vi "CONEX_SAG_control.vi"() -> ()   [LabVIEW 2016]
uses:
  <vilib>/Instr/_visa.llb/VISA Open Access Mode.ctl
panel:
  out "Actual Velocity [mm/s]":dbl
  out "write buffer":string
  in  "STOP":bool
  out "read buffer":string
  out "error out":errorcluster
  in  "error in (no error)":errorcluster
  in  "VISA resource name":refnum<visa-resource-name>="COM9"
  in  "Set new velocity":bool
  in  "Velocity [mm/s]":sgl=1.0
  in  "HOME":bool
  in  "Move Absolute":bool
  in  "Set Absolute Position":sgl=2.0
  in  "Move Relative":bool
  in  "Set Relative Position":sgl=1.0
  out "Current\nPosition\n[mm]":sgl=19.930592 format="%_8f"
  in  "stop code":bool
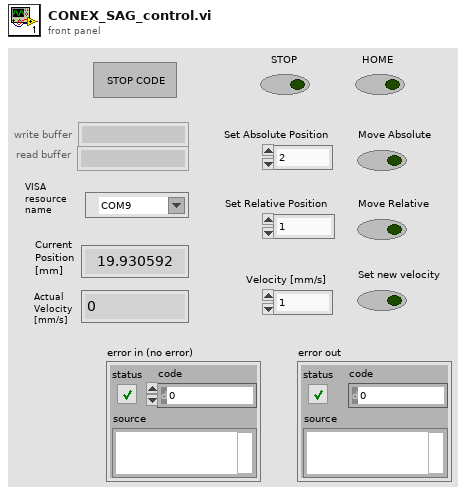
[diagram p1: front panel]
types:
  T1 = typedef "VISA Open Access Mode.ctl" = u32
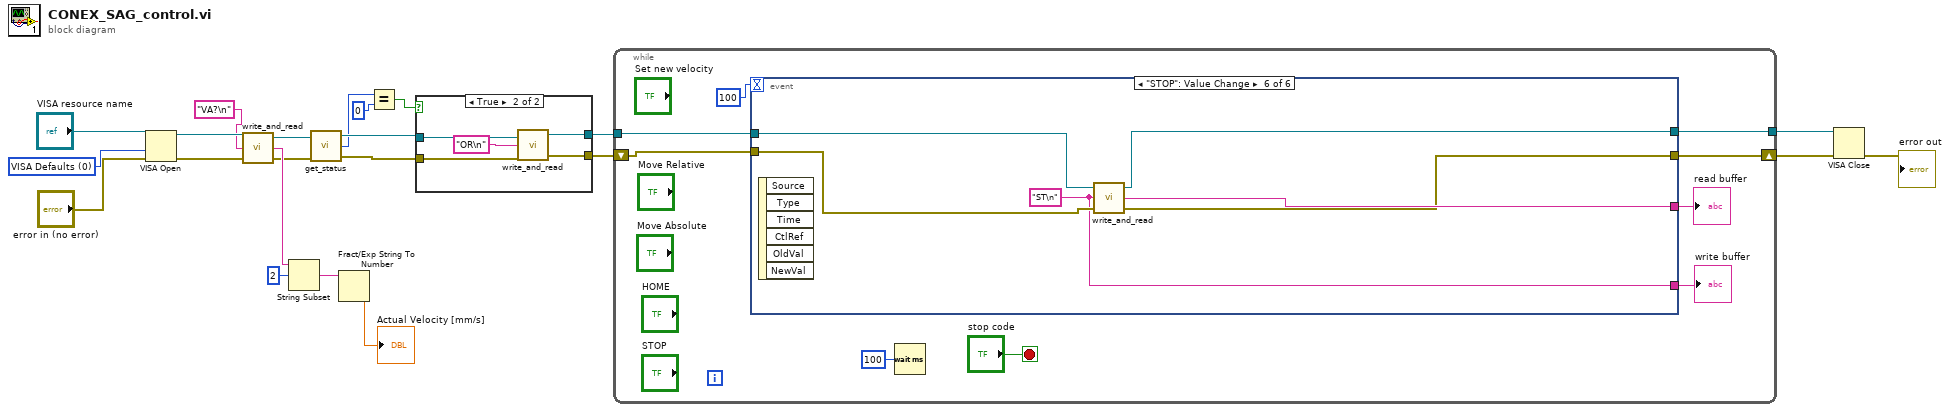
[diagram p0: block diagram]
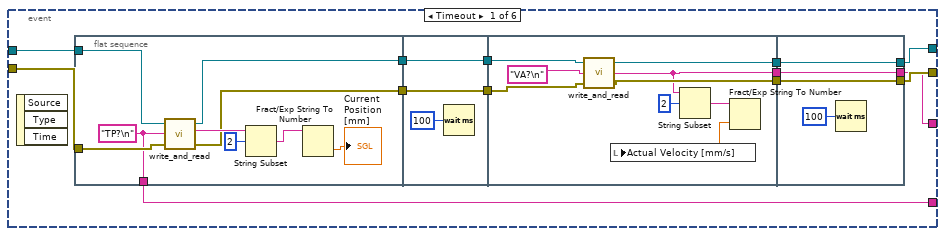
[diagram p3: hidden frame]
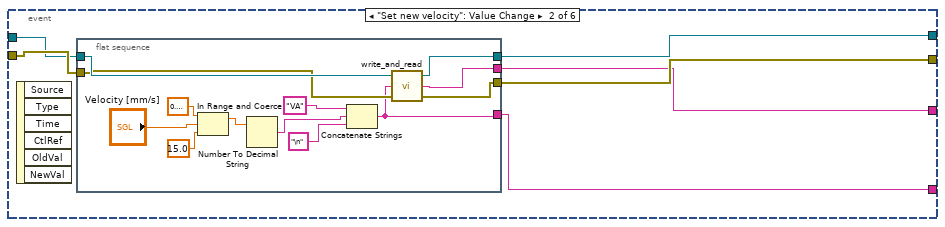
[diagram p4: hidden frame]
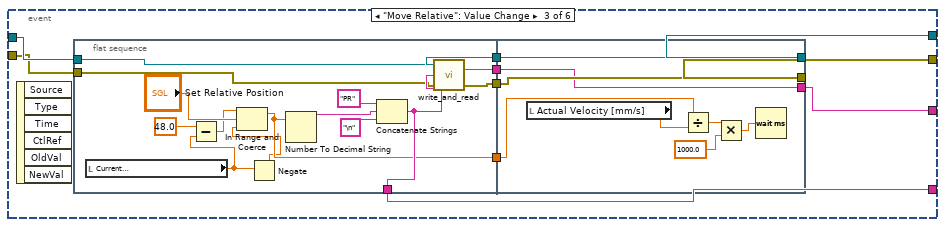
[diagram p5: hidden frame]
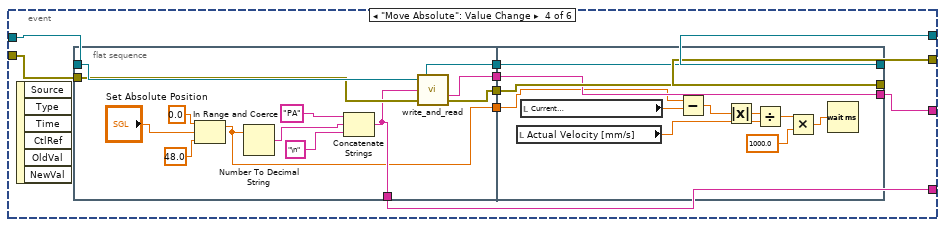
[diagram p6: hidden frame]
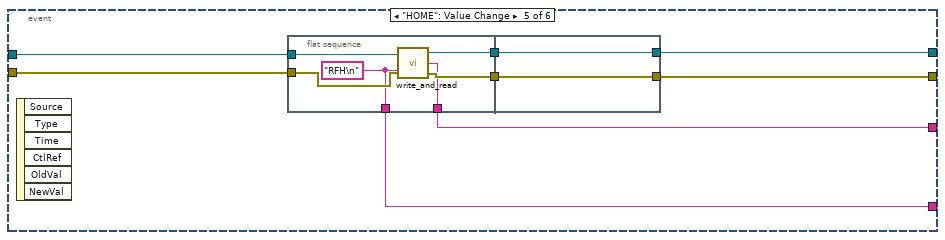
[diagram p7: hidden frame]
diagram:
  w20 = T1 0 items=["VISA Defaults"=0, "Exclusive Lock"=1, "Load Configured Settings"=4] ("Access Mode")
  n1 = VISA Open(access mode=w20, error in (no error)="error in (no error)", VISA resource name="VISA resource name") -> (VISA resource name=w16:refnum<visa-resource-name>, error out=w15:errorcluster)  [unwired: 2 in]
  n2 = call "write_and_read.vi"("error in"=w15, "write buffer"="VA?\n", "VISA resource name in"=w16) -> ("error out"=w6:errorcluster, "read buffer"=w12:string, "VISA resource name out"=w7:refnum<visa-resource-name>)
  n3 = String Subset(string=w12, offset (0)=2) -> (substring=w13:string)  [unwired: 1 in]
  n4 = call "get_status.vi"("VISA resource name in"=w7, "error in"=w6) -> ("VISA resource name out"=w5:refnum<visa-resource-name>, "Status"=w3:u8, "error out"=w4:errorcluster)
  n5 = Fract/Exp String To Number(string=w13) -> (number=→"Actual Velocity [mm/s]":dbl)  [unwired: 3 in, 1 out]
  n6 = Equal?(x=w3, y=u8 0) -> (x = y?=w1:bool)
  n7 = case shown="True" w1 {
    tunnel: [w24 w28] -> w9
    tunnel: [w23 w27] -> w8
    tunnel: w5 -> [w24 w26]
    tunnel: w4 -> [w23 w25]
    frame False {
    }
    frame True {
      n8 = call "write_and_read.vi"("error in"=w25, "write buffer"="OR\n", "VISA resource name in"=w26) -> ("error out"=w27:errorcluster, "VISA resource name out"=w28:refnum<visa-resource-name>)  [unwired: 1 out]
    }
  }
  n9 = while {
    shift-right: [w34] -> w18
    shift-left: w8 -> [w35]
    tunnel: w9 -> [w33]
    tunnel: [w32] -> w17
    stop <- "stop code" stop-if-true
    n10 = event shown="[5] \"STOP\": Value Change" {
      selector: _ -> [_ _ _ _ _ _]
      dyn-events: _ -> [_ _ _ _ _ _]
      timeout: 100 -> [_ _ _ _ _ _]
      tunnel: w35 -> [w50 w82 w101 w134 w169 w183]
      tunnel: [w43 w79 w99 w132 w167 w180] -> w34
      tunnel: w33 -> [w51 w81 w102 w135 w170 w184]
      tunnel: [w44 w80 w100 w133 w168 w182] -> w32
      tunnel: [w39 w78 w98 w131 w166 w181] -> w31
      tunnel: [w49 w77 w97 w130 w165 w179] -> w30
      event Timeout {
        n11 = event-data() -> ()  [unwired: 1 in, 3 out]
        n12 = flat-sequence {
          tunnel: w51 -> [w60]
          tunnel: w50 -> [w59]
          tunnel: [w54] -> w49
          tunnel: [w53] -> w48
          tunnel: [w52] -> w47
          tunnel: w48 -> [w63]
          tunnel: w47 -> [w62]
          tunnel: [w63] -> w46
          tunnel: [w62] -> w45
          tunnel: w46 -> [w69]
          tunnel: w45 -> [w68]
          tunnel: [w67] -> w42
          tunnel: [w66] -> w41
          tunnel: [w64] -> w40
          tunnel: [w75] -> w43
          tunnel: [w76] -> w44
          tunnel: w42 -> [w76]
          tunnel: w41 -> [w75]
          tunnel: w40 -> [w73]
          tunnel: [w73] -> w39
          frame #0 {
            w54 = "TP?\n"
            n13 = call "write_and_read.vi"("error in"=w59, "write buffer"=w54, "VISA resource name in"=w60) -> ("error out"=w52:errorcluster, "read buffer"=w58:string, "VISA resource name out"=w53:refnum<visa-resource-name>)
            n14 = String Subset(string=w58, offset (0)=2) -> (substring=w56:string)  [unwired: 1 in]
            n15 = Fract/Exp String To Number(string=w56) -> (number=→"Current\nPosition\n[mm]":dbl)  [unwired: 3 in, 1 out]
          }
          frame #1 {
            n16 = Wait (ms)(milliseconds to wait=u32 100) -> ()  [unwired: 1 out]
          }
          frame #2 {
            n17 = call "write_and_read.vi"("error in"=w68, "write buffer"="VA?\n", "VISA resource name in"=w69) -> ("error out"=w66:errorcluster, "read buffer"=w64:string, "VISA resource name out"=w67:refnum<visa-resource-name>)
            n18 = String Subset(string=w64, offset (0)=2) -> (substring=w71:string)  [unwired: 1 in]
            n19 = Fract/Exp String To Number(string=w71) -> (number=w72:dbl)  [unwired: 3 in, 1 out]
            n20 = local write "Actual Velocity [mm/s]"(w72) -> ()
          }
          frame #3 {
            n21 = Wait (ms)(milliseconds to wait=u32 100) -> ()  [unwired: 1 out]
          }
        }
      }
      event "Set new velocity": Value Change {
        n22 = event-data() -> ()  [unwired: 1 in, 6 out]
        n23 = flat-sequence {
          tunnel: w82 -> [w84]
          tunnel: w81 -> [w92]
          tunnel: [w83] -> w77
          tunnel: [w90] -> w80
          tunnel: [w89] -> w79
          tunnel: [w88] -> w78
          frame #0 {
            n24 = In Range and Coerce(upper limit=sgl 0.6, x="Velocity [mm/s]", lower limit=sgl 15.0) -> (coerced(x)=w87:sgl)  [unwired: 1 out]
            n25 = Number To Decimal String(number=w87) -> (decimal integer string=w86:string)  [unwired: 1 in]
            n26 = Concatenate Strings("VA" ("string"), w86, "\n" ("string")) -> (w83:string)
            n27 = call "write_and_read.vi"("error in"=w84, "write buffer"=w83, "VISA resource name in"=w92) -> ("error out"=w89:errorcluster, "read buffer"=w88:string, "VISA resource name out"=w90:refnum<visa-resource-name>)
          }
        }
      }
      event "Move Relative": Value Change {
        n28 = event-data() -> ()  [unwired: 1 in, 6 out]
        n29 = flat-sequence {
          tunnel: [w119] -> w105
          tunnel: [w118] -> w104
          tunnel: [w117] -> w103
          tunnel: w102 -> [w113]
          tunnel: w101 -> [w112]
          tunnel: [w111] -> w97
          tunnel: [w110] -> w96
          tunnel: [w128] -> w100
          tunnel: w105 -> [w128]
          tunnel: w104 -> [w127]
          tunnel: [w127] -> w99
          tunnel: [w126] -> w98
          tunnel: w103 -> [w126]
          tunnel: w96 -> [w125]
          frame #0 {
            n30 = local read "Current\nPosition\n[mm]"() -> (w107:sgl)
            n31 = Subtract(x=48.0, y=w107) -> (x-y=w106:dbl)
            n32 = Negate(x=w107) -> (-x=w109:sgl)
            n33 = In Range and Coerce(upper limit=w106, x="Set Relative Position", lower limit=w109) -> (coerced(x)=w110:dbl)  [unwired: 1 out]
            n34 = Number To Decimal String(number=w110) -> (decimal integer string=w116:string)  [unwired: 1 in]
            n35 = Concatenate Strings("PR" ("string"), w116, "\n" ("string")) -> (w111:string)
            n36 = call "write_and_read.vi"("error in"=w112, "write buffer"=w111, "VISA resource name in"=w113) -> ("error out"=w118:errorcluster, "read buffer"=w117:string, "VISA resource name out"=w119:refnum<visa-resource-name>)
          }
          frame #1 {
            n37 = local read "Actual Velocity [mm/s]"() -> (w124:dbl)
            n38 = Divide(x=w125, y=w124) -> (x/y=w123:dbl)
            n39 = Multiply(x=w123, y=sgl 1000.0) -> (x*y=w121:dbl)
            n40 = Wait (ms)(milliseconds to wait=w121) -> ()  [unwired: 1 out]
          }
        }
      }
      event "Move Absolute": Value Change {
        n41 = event-data() -> ()  [unwired: 1 in, 6 out]
        n42 = flat-sequence {
          tunnel: [w148] -> w138
          tunnel: [w147] -> w137
          tunnel: [w146] -> w136
          tunnel: w135 -> [w142]
          tunnel: w134 -> [w141]
          tunnel: [w140] -> w130
          tunnel: [w139] -> w129
          tunnel: [w162] -> w133
          tunnel: w138 -> [w162]
          tunnel: w137 -> [w161]
          tunnel: [w161] -> w132
          tunnel: [w160] -> w131
          tunnel: w136 -> [w160]
          tunnel: w129 -> [w154]
          frame #0 {
            n43 = In Range and Coerce(upper limit=sgl 0.0, x="Set Absolute Position", lower limit=sgl 48.0) -> (coerced(x)=w139:sgl)  [unwired: 1 out]
            n44 = Number To Decimal String(number=w139) -> (decimal integer string=w145:string)  [unwired: 1 in]
            n45 = Concatenate Strings("PA" ("string"), w145, "\n" ("string")) -> (w140:string)
            n46 = call "write_and_read.vi"("error in"=w141, "write buffer"=w140, "VISA resource name in"=w142) -> ("error out"=w147:errorcluster, "read buffer"=w146:string, "VISA resource name out"=w148:refnum<visa-resource-name>)
          }
          frame #1 {
            n47 = local read "Actual Velocity [mm/s]"() -> (w156:dbl)
            n48 = local read "Current\nPosition\n[mm]"() -> (w155:sgl)
            n49 = Subtract(x=w154, y=w155) -> (x-y=w153:sgl)
            n50 = Absolute Value(x=w153) -> (abs(x)=w152:sgl)
            n51 = Divide(x=w152, y=w156) -> (x/y=w159:dbl)
            n52 = Multiply(x=w159, y=sgl 1000.0) -> (x*y=w157:dbl)
            n53 = Wait (ms)(milliseconds to wait=w157) -> ()  [unwired: 1 out]
          }
        }
      }
      event "HOME": Value Change {
        n54 = event-data() -> ()  [unwired: 1 in, 6 out]
        n55 = flat-sequence {
          tunnel: w170 -> [w176]
          tunnel: w169 -> [w175]
          tunnel: [w172] -> w166
          tunnel: [w171] -> w165
          tunnel: [w174] -> w164
          tunnel: [w173] -> w163
          tunnel: [w177] -> w167
          tunnel: [w178] -> w168
          tunnel: w164 -> [w178]
          tunnel: w163 -> [w177]
          frame #0 {
            w171 = "RFH\n" ("string")
            n56 = call "write_and_read.vi"("error in"=w175, "write buffer"=w171, "VISA resource name in"=w176) -> ("error out"=w173:errorcluster, "read buffer"=w172:string, "VISA resource name out"=w174:refnum<visa-resource-name>)
          }
          frame #1 {
          }
        }
      }
      event "STOP": Value Change {
        w179 = "ST\n" ("string")
        n57 = event-data() -> ()  [unwired: 1 in, 6 out]
        n58 = call "write_and_read.vi"("error in"=w183, "write buffer"=w179, "VISA resource name in"=w184) -> ("error out"=w180:errorcluster, "read buffer"=w181:string, "VISA resource name out"=w182:refnum<visa-resource-name>)
      }
    }
    "read buffer" <- w31
    "write buffer" <- w30
    n59 = Wait (ms)(milliseconds to wait=u32 100) -> ()  [unwired: 1 out]
  }
  n60 = VISA Close(VISA resource name=w17, error in (no error)=w18) -> (error out=→"error out":errorcluster)
